vi "RoboDAQ7.vi"() -> ()   [LabVIEW 2015]
uses:
  Default file name.vi
  <vilib>/Instr/_visa.llb/VISA Configure Serial Port (Instr).vi
  GlobalVISA7.vi
  GlobalIODataSize7.vi
  GlobalNumPlotChannels.vi
  GlobalNumPlotPoints.vi
  GlobalDataPath7.vi
  GlobalDataSize.vi
  GlobalParamSize.vi
  GlobalErrorCAN_ID.vi
  GlobalInitialParamVals.vi
  GlobalDataNum.vi
  GlobalDataNames.vi
  GlobalDataFileRefnum7.vi
  GlobalLabVIEWStart.vi
panel:
  in  "Flow control\n0 = none\n2 = RTS/CTS\n(hardware)":i16=2 min=0 max=5 step=1
  in  "Default file base name":string="Test"
  in  "Baud Rate":i32=460800
  in  "VISA resource name":refnum<visa-resource-name>="COM6"
  # "To use the serial  port:\n- comment the #IFNDEF in the software.h corresponding to blue tooth.\n- restart lab view with baud rate: 921600, flow control 0, VISA resource as COM-10 (this may change, \n but right now its the port right next to the mic jack)\n- make sure the blue tooth box is disconnected. \n\ntouse the blue tooth: (default)\n- comment the #IFNDEF line in software.h corresponding to serial port\n- restart lab view with baud rate 460800, flow control 2, VISA rosource COM-6 (this may change)"
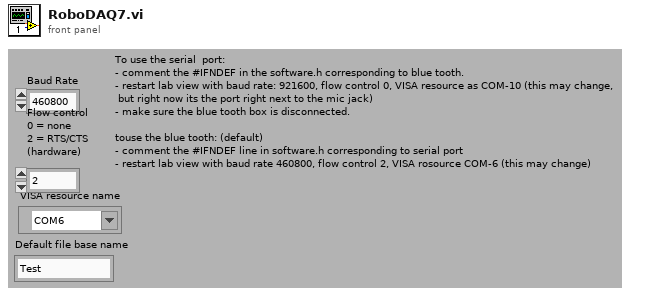
[diagram p1: front panel]
types:
  T1 = cluster{"ERROR CHANNELS":dbl[], "Error Boards":string[]}
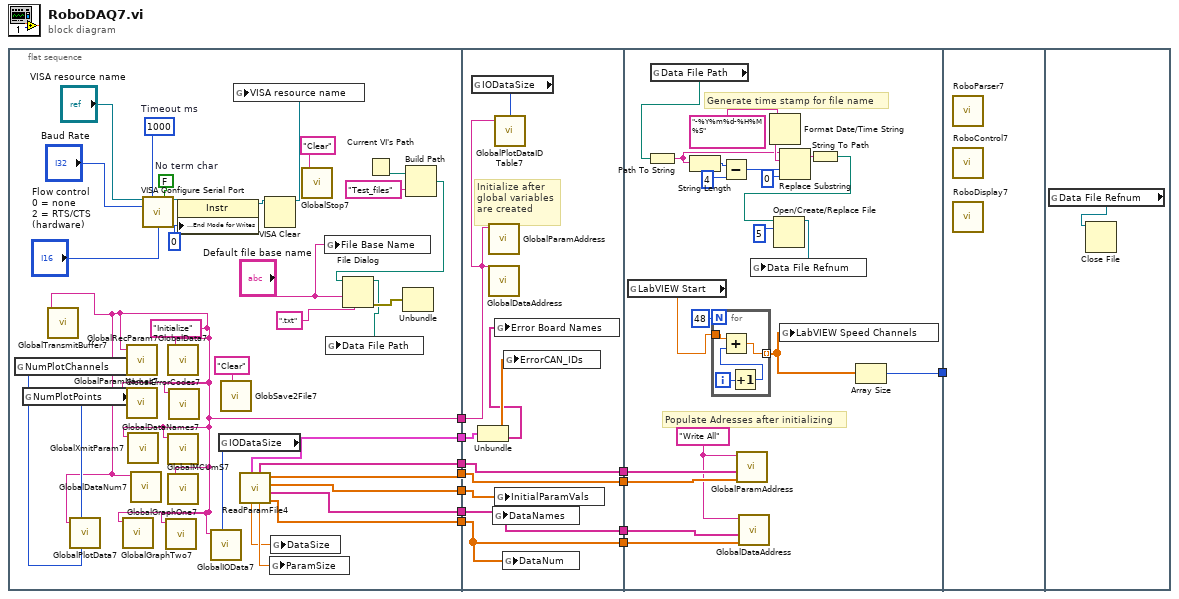
[diagram p0: block diagram]
diagram:
  n1 = flat-sequence {
    tunnel: [w30] -> w12
    tunnel: [w29] -> w11
    tunnel: [w28] -> w10
    tunnel: [w27] -> w9
    tunnel: [w22] -> w8
    tunnel: [w19] -> w3
    tunnel: [w17] -> w2
    tunnel: w12 -> [w45]
    tunnel: w11 -> [w50]
    tunnel: w10 -> [w44]
    tunnel: w9 -> [w43]
    tunnel: w8 -> [w52]
    tunnel: [w45] -> w7
    tunnel: [w50] -> w6
    tunnel: [w43] -> w5
    tunnel: [w44] -> w4
    tunnel: w3 -> [w49]
    tunnel: w2 -> [w48]
    tunnel: w4 -> [w70]
    tunnel: w5 -> [w71]
    tunnel: w6 -> [w72]
    tunnel: w7 -> [w73]
    tunnel: [w54] -> w1
    tunnel: w1 -> [_]
    frame #0 {
      w22 = "Initialize"
      w40 = 1000  # Timeout ms
      w41 = FALSE  # No term char
      n2 = global read "GlobalNumPlotChannels.vi" "NumPlotChannels"() -> (w23:i32)
      n3 = global read "GlobalNumPlotPoints.vi" "NumPlotPoints"() -> (w24:i32)
      n4 = call "GlobalTransmitBuffer7.vi"("Function select"=w22) -> ()  [unwired: 2 in, 3 out]
      n5 = call "GlobalPlotData7.vi"("Function select"=w22, "# Plot points"=w24, "# Data channels"=w23) -> ()  [unwired: 2 in, 1 out]
      n6 = call "GlobalGraphTwo7.vi"("Function select"=w22) -> ()  [unwired: 3 in, 2 out]
      n7 = call "GlobalRecParam7.vi"("Function select"=w22) -> ()  [unwired: 2 in, 1 out]
      n8 = call "GlobalParamNames7.vi"("Function select"=w22) -> ()  [unwired: 3 in, 1 out]
      n9 = call "GlobalXmitParam7.vi"("Function select"=w22) -> ()  [unwired: 3 in, 1 out]
      n10 = call "GlobalDataNum7.vi"("Function select"=w22) -> ()  [unwired: 3 in, 2 out]
      n11 = call-poly "VISA Configure Serial Port"("VISA resource name"="VISA resource name", "timeout (10sec)"=w40, "Enable Termination\nChar (T)"=w41, "baud rate (9600)"="Baud Rate", "flow control (0:none)"="Flow control\n0 = none\n2 = RTS/CTS\n(hardware)") -> ("VISA resource name out"=w35:refnum<visa-resource-name>)  [unwired: 9 in, 1 out]
      n12 = call "GlobalGraphOne7.vi"("Function select"=w22) -> ()  [unwired: 3 in, 2 out]
      n13 = call "GlobalData7.vi"("Function select"=w22) -> ()  [unwired: 2 in, 3 out]
      n14 = call "GlobalDataNames7.vi"("Function select"=w22) -> ()  [unwired: 3 in, 2 out]
      n15 = call "GlobalMCUmS7.vi"("Function select"=w22) -> ()  [unwired: 1 in, 2 out]
      n16 = call "GlobalErrorCodes7.vi"("Function select"=w22) -> ()  [unwired: 3 in, 4 out]
      n17 = property class="Instr"(reference=w35, "Serial Settings:End Mode for Writes"=0) -> (reference out=w34:refnum<visa-resource-name>)  [unwired: 1 in, 1 out]
      n18 = global read "GlobalIODataSize7.vi" "IODataSize"() -> (w21:i32)
      n19 = call "GlobalIOData7.vi"("Function select"=w22, "IO points array size"=w21) -> ()  [unwired: 3 in, 2 out]
      n20 = call "GlobSave2File7.vi"("Function select"="Clear") -> ()  [unwired: 1 out]
      n21 = call "ReadParamFile4.vi"() -> ("Data #"=w27:dbl[], "Data Name"=w28:string[], "Param Val"=w19:dbl[], "Param #"=w29:dbl[], "Param Size"=w31:dbl, "Param Name"=w30:string[], "Data Size"=w26:dbl, "Error Cluster"=w17:T1)  [unwired: 4 in]
      n22 = VISA Clear(VISA resource name=w34) -> (VISA resource name out=w38:refnum<visa-resource-name>)  [unwired: 1 in, 1 out]
      n23 = global write "GlobalVISA7.vi" "VISA resource name"(w38) -> ()
      n24 = global write "GlobalParamSize.vi" "ParamSize"(w31) -> ()
      n25 = global write "GlobalDataSize.vi" "DataSize"(w26) -> ()
      n26 = call "GlobalStop7.vi"("Function select"="Clear") -> ()  [unwired: 1 out]
      n27 = global write "Default file name.vi" "File Base Name"("Default file base name") -> ()
      n28 = Current VI's Path() -> (path=w16:path)
      n29 = Build Path(base path=w16, name or relative path="Test_files") -> (appended path=w14:path)
      n30 = File Dialog(6:".txt", 9:"Default file base name", 11:w14) -> (0:w32:errorcluster, 3:w20:path)  [unwired: 4 in, 2 out]
      n31 = global write "GlobalDataPath7.vi" "Data File Path"(w20) -> ()
      n32 = Unbundle(w32) -> ()  [unwired: 3 out]
    }
    frame #1 {
      # "Initialize after\nglobal variables\nare created"
      n33 = global read "GlobalIODataSize7.vi" "IODataSize"() -> (w51:i32)
      n34 = Unbundle(w48) -> ("ERROR CHANNELS"=w47:dbl[], "Error Boards"=w46:string[])
      n35 = call "GlobalParamAddress.vi"("Function select"=w52) -> ()  [unwired: 3 in, 4 out]
      n36 = call "GlobalDataAddress.vi"("Function select"=w52) -> ()  [unwired: 3 in, 4 out]
      n37 = global write "GlobalDataNames.vi" "DataNames"(w44) -> ()
      n38 = call "GlobalPlotDataIDTable7.vi"("IO points array size"=w51, "Function select"=w52) -> ()  [unwired: 2 in, 1 out]
      n39 = global write "GlobalErrorCAN_ID.vi" "Error Board Names"(w46) -> ()
      n40 = global write "GlobalInitialParamVals.vi" "InitialParamVals"(w49) -> ()
      n41 = global write "GlobalDataNum.vi" "DataNum"(w43) -> ()
      n42 = global write "GlobalErrorCAN_ID.vi" "ErrorCAN_IDs"(w47) -> ()
    }
    frame #2 {
      w69 = "Write All"
      # "Populate Adresses after initializing"
      # "Generate time stamp for file name"
      n43 = global read "GlobalLabVIEWStart.vi" "LabVIEW Start"() -> (w53:dbl)
      n44 = global read "GlobalDataPath7.vi" "Data File Path"() -> (w58:path)
      n45 = Path To String(path=w58) -> (string=w59:string)
      n46 = String Length(string=w59) -> (length=w66:i32)
      n47 = for {
        N: 48 -> [_]
        tunnel: [w74] -> w55 mode=indexing
        tunnel: w53 -> [w77]
        i -> [w76]
        n48 = Increment(x=w76) -> (x+1=w75:i32)
        n49 = Add(x=w77, y=w75) -> (x+y=w74:dbl)
      }
      n50 = Subtract(x=w66, y=4) -> (x-y=w64:i32)
      n51 = call "GlobalParamAddress.vi"("Parameter ID In"=w72, "Parameter Names In"=w73, "Function select"=w69) -> ()  [unwired: 1 in, 4 out]
      n52 = call "GlobalDataAddress.vi"("Data IDs In"=w71, "Data Names In"=w70, "Function select"=w69) -> ()  [unwired: 1 in, 4 out]
      n53 = Format Date/Time String(time format string (%c)="-%Y%m%d-%H%M%S") -> (date/time string=w60:string)  [unwired: 2 in]
      n54 = Replace Substring(2:0, 3:w64, 4:w60, 5:w59) -> (1:w62:string)  [unwired: 1 out]
      n55 = global write "GlobalLabVIEWStart.vi" "LabVIEW Speed Channels"(w55) -> ()
      n56 = String To Path(string=w62) -> (path=w57:path)
      n57 = Open/Create/Replace File(file path (use dialog)=w57, operation (0:open)=5) -> (refnum out=w67:refnum<file>)  [unwired: 4 in, 2 out]
      n58 = global write "GlobalDataFileRefnum7.vi" "Data File Refnum"(w67) -> ()
      n59 = Array Size(array=w55) -> (size(s)=w54:i32)
    }
    frame #3 {
      n60 = call "RoboParser7.vi"() -> ()  [unwired: 1 in]
      n61 = call "RoboControl7.vi"() -> ()  [unwired: 1 in]
      n62 = call "RoboDisplay7.vi"() -> ()  [unwired: 1 in]
    }
    frame #4 {
      n63 = global read "GlobalDataFileRefnum7.vi" "Data File Refnum"() -> (w78:refnum<file>)
      n64 = Close File(refnum=w78) -> ()  [unwired: 1 in, 2 out]
    }
  }
